vi "CLSUIP_CenterOnPoint.vi"(1 "error in (no error)":errorcluster, 2 "Position":cluster{"x":i32, "y":i32}, 3 "CtrlTerm Refnum":refnum<vi>) -> (0 "error out":errorcluster)   [LabVIEW 2021, in "MemberVICreation.lvlib" / "VIRetooler.lvclass"]
uses:
  <resource>/Framework/Providers/LVClassLibrary/NewAccessors/VIRetooler/VIRetooler.lvclass
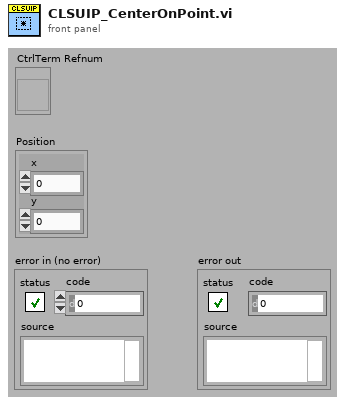
[diagram p1: front panel]
types:
  T1 = typedef "LVRectTypeDef.ctl" = cluster{"left":i16, "top":i16, "right":i16, "bottom":i16}
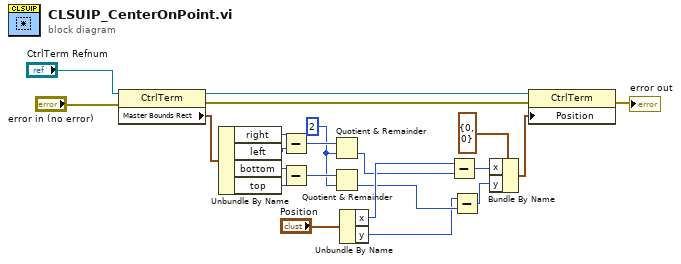
[diagram p0: block diagram]
diagram:
  w12 = i16 2 ("y")
  n1 = property class="CtrlTerm"(reference="CtrlTerm Refnum", error in="error in (no error)") -> (reference out=w20:refnum<vi>, error out=w19:errorcluster, "Master Bounds Rect"=w18:T1)
  n2 = Unbundle By Name(w18) -> ("right"=w17:i16, "left"=w11:i16, "bottom"=w15:i16, "top"=w16:i16)
  n3 = Subtract(x=w17, y=w11) -> (x-y=w14:i16)
  n4 = Subtract(x=w15, y=w16) -> (x-y=w13:i16)
  n5 = Quotient & Remainder(x=w14, y=w12) -> (floor(x/y)=w8:i16)  [unwired: 1 out]
  n6 = Quotient & Remainder(x=w13, y=w12) -> (floor(x/y)=w7:i16)  [unwired: 1 out]
  n7 = Unbundle By Name("Position") -> ("x"=w9:i32, "y"=w6:i32)
  n8 = Subtract(x=w9, y=w8) -> (x-y=w4:i32)
  n9 = Subtract(x=w6, y=w7) -> (x-y=w3:i32)
  n10 = Bundle By Name(cluster=cluster{"x":i32, "y":i32} {"x"=0, "y"=0} ("Position"), "x"=w4, "y"=w3) -> (w2:cluster{"x":i32, "y":i32})
  n11 = property class="CtrlTerm"(reference=w20, error in=w19, "Position"=w2) -> (error out=→"error out":errorcluster)  [unwired: 1 out]
